vi "Mp285Control.vi"() -> ()   [LabVIEW 2010]
uses:
  james/LabView/AOD_Control/SerialController/Serial Controller.lvclass
panel:
  in  "Set Relative":bool
  in  "Absolute":bool caption="Relative"
  in  "Run":bool
  in  "Anterior":bool
  in  "Posterior":bool
  in  "Right":bool
  in  "Left":bool
  in  "Up":bool
  in  "Down":bool
  out "X                  Y                 Z":dbl[](array[numeric])=[0.0, 0.0, 5.0] caption="Absolute Position"
  in  "Step (mm)":dbl
  # "Position"
  # "Motor Control"
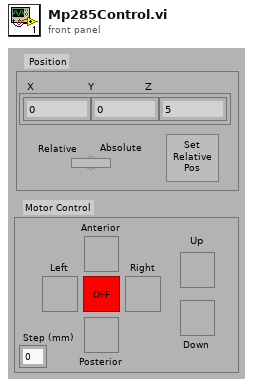
[diagram p1: front panel]
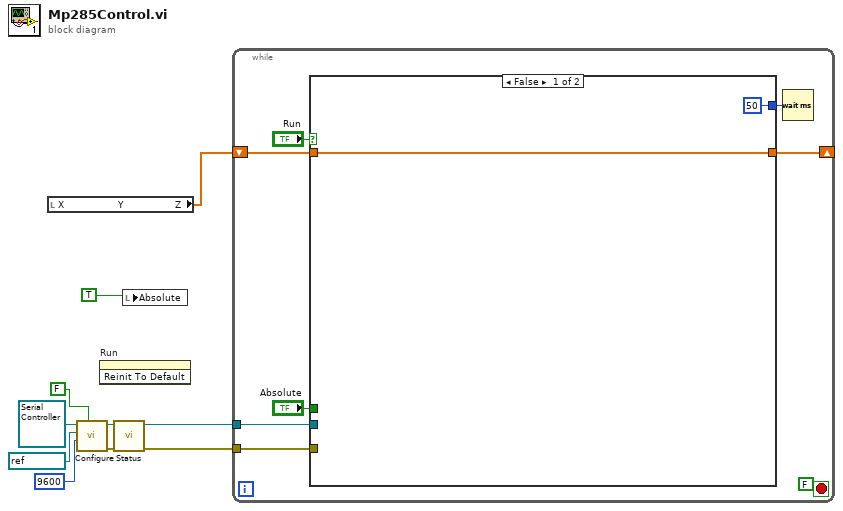
[diagram p0: block diagram]
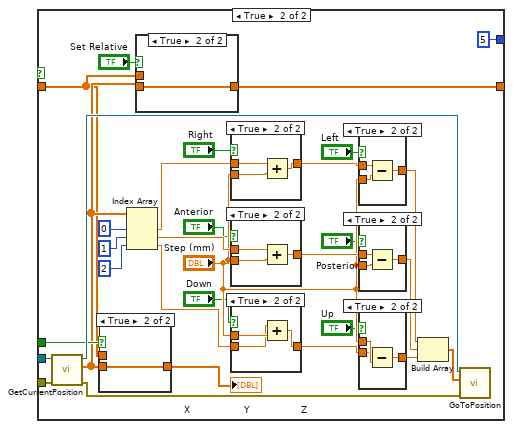
[diagram p2: hidden frame]
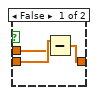
[diagram p4: hidden frame]
diagram:
  n1 = local read "X                  Y                 Z"() -> (w2:dbl[])
  n2 = call-dynamic "Configure.vi"("Reset"=FALSE, "baud rate (9600)"=u32 9600, "VISA resource name"=refnum<visa-resource-name> "COM2", "Serial Controller in"=refnum<class "Serial Controller.lvclass"> refnum) -> ("error out"=w7:errorcluster, "Serial Controller out"=w8:refnum<class "Serial Controller.lvclass">)  [unwired: 6 in]
  n3 = invoke on="Run" class="Bool (strict)" method="Reinit To Default"() -> ()  [unwired: 3 in, 3 out]
  n4 = call-dynamic "Status.vi"("error in (no error)"=w7, "Serial Controller in"=w8) -> ("error out"=w9:errorcluster, "Serial Controller out"=w10:refnum<class "Serial Controller.lvclass">)  [unwired: 7 in, 1 out]
  n5 = local write "Absolute"(TRUE) -> ()
  n6 = while {
    tunnel: w10 -> [w18]
    tunnel: w9 -> [w17]
    shift-right: [w11] -> _
    shift-left: w2 -> [w12]
    stop <- FALSE stop-if-true
    n7 = case shown="False" "Run" {
      tunnel: w18 -> [_ w51]
      tunnel: w17 -> [_ w50]
      tunnel: [50 u32 5 ("milliseconds to wait")] -> w16
      tunnel: "Absolute" -> [_ w25]
      tunnel: w12 -> [w19 w21]
      tunnel: [w19 w23] -> w11
      frame False {
      }
      frame True {
        n8 = call-dynamic "GetCurrentPosition.vi"("error in (no error)"=w50, "Serial Controller in"=w51) -> ("error out"=w49:errorcluster, "Position"=w22:dbl[], "Serial Controller out"=w48:refnum<class "Serial Controller.lvclass">)  [unwired: 7 in]
        n9 = case shown="True" w25 {
          tunnel: w22 -> [w55 w57]
          tunnel: [w56 w57] -> w26
          tunnel: w21 -> [w54 _]
          frame False {
            n10 = Subtract(x=w55, y=w54) -> (x-y=w56:dbl[])
          }
          frame True {
          }
        }
        "X                  Y                 Z" <- w26
        n11 = Index Array(array=w22, index #1=0 ("index"), index #2=1 ("index"), index #3=2 ("index")) -> (element #1=w43:dbl, element #2=w42:dbl, element #3=w41:dbl)
        n12 = case shown="True" "Set Relative" {
          tunnel: w21 -> [w52 _]
          tunnel: [w52 w53] -> w23
          tunnel: w22 -> [_ w53]
          frame False {
          }
          frame True {
          }
        }
        n13 = case shown="True" "Right" {
          tunnel: w43 -> [w78 w80]
          tunnel: [w78 w79] -> w40
          tunnel: "Step (mm)" -> [_ w81]
          frame False {
          }
          frame True {
            n14 = Add(x=w80, y=w81) -> (x+y=w79:dbl)
          }
        }
        n15 = case shown="True" "Anterior" {
          tunnel: w42 -> [w74 w76]
          tunnel: [w74 w75] -> w39
          tunnel: "Step (mm)" -> [_ w77]
          frame False {
          }
          frame True {
            n16 = Add(x=w76, y=w77) -> (x+y=w75:dbl)
          }
        }
        n17 = case shown="True" "Down" {
          tunnel: w41 -> [w70 w72]
          tunnel: [w70 w71] -> w38
          tunnel: "Step (mm)" -> [_ w73]
          frame False {
          }
          frame True {
            n18 = Add(x=w72, y=w73) -> (x+y=w71:dbl)
          }
        }
        n19 = case shown="True" "Left" {
          tunnel: [w66 w67] -> w37
          tunnel: w40 -> [w66 w68]
          tunnel: "Step (mm)" -> [_ w69]
          frame False {
          }
          frame True {
            n20 = Subtract(x=w68, y=w69) -> (x-y=w67:dbl)
          }
        }
        n21 = case shown="True" "Posterior" {
          tunnel: [w62 w65] -> w36
          tunnel: w39 -> [w62 w63]
          tunnel: "Step (mm)" -> [_ w64]
          frame False {
          }
          frame True {
            n22 = Subtract(x=w63, y=w64) -> (x-y=w65:dbl)
          }
        }
        n23 = case shown="True" "Up" {
          tunnel: [w58 w59] -> w35
          tunnel: w38 -> [w58 w60]
          tunnel: "Step (mm)" -> [_ w61]
          frame False {
          }
          frame True {
            n24 = Subtract(x=w60, y=w61) -> (x-y=w59:dbl)
          }
        }
        n25 = Build Array(w37, w36, w35) -> (w34:dbl[])
        n26 = call-dynamic "GoToPosition.vi"("error in (no error)"=w49, "Position"=w34, "Serial Controller in"=w48) -> ()  [unwired: 7 in, 2 out]
      }
    }
    n27 = Wait (ms)(milliseconds to wait=w16) -> ()  [unwired: 1 out]
  }
